vi "Setup manipulator (SubVI).vi"(0 "Release?":bool, 1 "G_upper bound":i32, 3 "M_lower bound":i32, 11 "error in (no error)":errorcluster, 12 "M_Encoder Ref In":T1, 14 "G_Encoder Ref In":T1) -> (15 "error out":errorcluster)   [LabVIEW 2017]
uses:
  <vilib>/myRIO/Instrument Drivers/Onboard IO/Encoder/typedefs/Encoder Reference.ctl
  <vilib>/myRIO/Common/Instrument Driver Framework/Utilities/typedefs/myRIO Generic Hardware Reference.ctl
  <vilib>/myRIO/Common/Instrument Driver Framework/Utilities/typedefs/Hardware Version Enum.ctl
  <vilib>/myRIO/Common/Instrument Driver Framework/Utilities/typedefs/myRIO v1.0 Reference.ctl
  <vilib>/myRIO/Common/Instrument Driver Framework/Utilities/typedefs/Generic FPGA Reference.ctl
  <vilib>/myRIO/Common/Instrument Driver Framework/myRIO v1.0/Encoder/typedefs/Encoder Channels Enum.ctl
  <vilib>/myRIO/Instrument Drivers/Onboard IO/DIO/typedefs/DIO Reference.ctl
  <vilib>/myRIO/Common/Instrument Driver Framework/myRIO v1.0/DIO/typedefs/DIO Channels List.ctl
  <vilib>/myRIO/Common/Instrument Driver Framework/myRIO v1.0/DIO/typedefs/DIO Channels Enum.ctl
  <vilib>/userdefined/High Color/nirio_resource_hc.ctl
  <vilib>/myRIO/Common/Instrument Driver Framework/Utilities/vis/Is FPGA Ref Available.vi
  <vilib>/myRIO/Common/Instrument Driver Framework/myRIO v1.0/DIO/vis/myRIO v1.1 Open DIO.vi
  <vilib>/myRIO/Instrument Drivers/Onboard IO/DIO/vis/Write.vi
  <vilib>/myRIO/Common/Instrument Driver Framework/Utilities/vis/Validate Channels.vi
  <vilib>/myRIO/Common/Instrument Driver Framework/myRIO v1.0/DIO/vis/myRIO v1.0 Reserve DIO.vi
  <vilib>/myRIO/Common/Instrument Driver Framework/myRIO v1.0/Resource Manager/vis/myRIO v1.0 Reserve Channel List.vi
  <vilib>/myRIO/Common/Instrument Driver Framework/myRIO v1.0/DIO/vis/myRIO v1.0 Build MUX Configuration DIO.vi
  <vilib>/myRIO/Common/Instrument Driver Framework/myRIO v1.0/Resource Manager/vis/myRIO v1.0 Reserve Channel.vi
  <vilib>/myRIO/Common/Instrument Driver Framework/myRIO v1.0/Resource Manager/vis/myRIO v1.0 Unreserve Channel.vi
  <vilib>/myRIO/Common/Instrument Driver Framework/myRIO v1.0/Resource Manager/vis/myRIO v1.0 Create Configuration List.vi
  <vilib>/myRIO/Common/Instrument Driver Framework/myRIO v1.0/Resource Manager/vis/myRIO v1.0 Build Mutex Name.vi
  <vilib>/Utility/error.llb/Error Cluster From Error Code.vi
  <vilib>/myRIO/Common/Instrument Driver Framework/myRIO v1.0/Encoder/vis/myRIO v1.0 Read Encoder.vi
  <vilib>/Utility/VariantDataType/GetNumericInfo.vi
  <vilib>/myRIO/Common/Instrument Driver Framework/myRIO v1.0/myRIO v1.1 Open.vi
  <vilib>/myRIO/Common/Instrument Driver Framework/Utilities/vis/IO Manager.vi
  <vilib>/myRIO/Common/Instrument Driver Framework/Utilities/vis/Configuration Manager.vi
  <vilib>/myRIO/Common/Instrument Driver Framework/myRIO v1.0/Resource Manager/vis/myRIO v1.0 Configure IO.vi
  <vilib>/myRIO/Common/Instrument Driver Framework/myRIO v1.0/myRIO v1.0 Close.vi
  <vilib>/myRIO/Common/Instrument Driver Framework/myRIO v1.0/DIO/vis/myRIO v1.0 Write DIO.vi
  <vilib>/myRIO/Express VI/Onboard IO/DO/DO Express VI.xnode
  <vilib>/myRIO/Instrument Drivers/Onboard IO/DIO/vis/myRIO DIO Open.xnode
  <vilib>/myRIO/Instrument Drivers/Onboard IO/Encoder/Encoder.lvlib
  <vilib>/myRIO/Instrument Drivers/Onboard IO/DIO/DIO.lvlib
panel:
  in  "stopG":bool
  out "G+":bool
  out "G enc val":i32
  out "M+":bool
  in  "stopM":bool
  out "M enc val":i32
  # "SET UP THE VALUES"
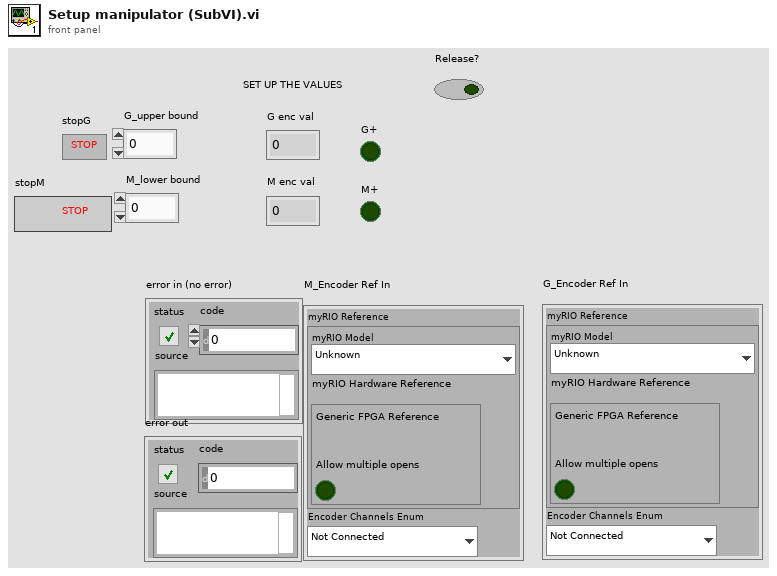
[diagram p1: front panel]
types:
  T1 = typedef "Encoder.lvlib/Encoder Reference.ctl" = cluster{"myRIO Reference":T2, "Encoder Channels Enum":T6}
  T2 = typedef "myRIO Generic Hardware Reference.ctl" = cluster{"myRIO Model":T3, "myRIO Hardware Reference":T4}
  T3 = typedef "Hardware Version Enum.ctl" = enum16{"Unknown", "myRIO-1900", "myRIO-1950", "roboRIO", "NI ELVIS RIO CM"}
  T4 = typedef "myRIO v1.0 Reference.ctl" = cluster{"Generic FPGA Reference":T5, "Allow multiple opens":bool}
  T5 = typedef "Generic FPGA Reference.ctl" = refnum<k20>
  T6 = typedef "Encoder Channels Enum.ctl" = enum16{"Not Connected", "C/ENC0", "C/ENC1", "A/ENC", "B/ENC", "DIO/ENC0", "DIO/ENC1", "DIO/ENC2", "DIO/ENC3", "DIO/ENC4"}
  T7 = typedef "DIO.lvlib/DIO Reference.ctl" = cluster{"myRIO Reference":T2, "DIO Channels List":T8}
  T8 = typedef "DIO Channels List.ctl" = T9[]
  T9 = typedef "DIO Channels Enum.ctl" = enum16{"Not Connected", "C/DIO0", "C/DIO1", "C/DIO2", "C/DIO3", "C/DIO4", "C/DIO5", "C/DIO6", "C/DIO7", "A/DIO0", "A/DIO1", "A/DIO2", "A/DIO3", "A/DIO4", "A/DIO5", "A/DIO6", "A/DIO7", "A/DIO8", "A/DIO9", "A/DIO10", "A/DIO11", "A/DIO12", "A/DIO13", "A/DIO14", "A/DIO15", "B/DIO0", "B/DIO1", "B/DIO2", "B/DIO3", "B/DIO4", "B/DIO5", "B/DIO6", "B/DIO7", "B/DIO8", "B/DIO9", "B/DIO10", "B/DIO11", "B/DIO12", "B/DIO13", "B/DIO14", "B/DIO15", "LED0", "LED1", "LED2", "LED3", "Button0", "DIO/DIO0", "DIO/DIO1", "DIO/DIO2", "DIO/DIO3", "DIO/DIO4", "DIO/DIO5", "DIO/DIO6", "DIO/DIO7", "DIO/DIO8", "DIO/DIO9", "SPI/CS0", "SPI/CS1", "SPI/CS2", "SPI/CS3", "LED RADIO (Green)", "LED RADIO (Red)", "LED COMM (Green)", "LED COMM (Red)", "LED MODE (Green)", "LED MODE (Red)"}
  T10 = typedef "nirio_resource_hc.ctl" = tag
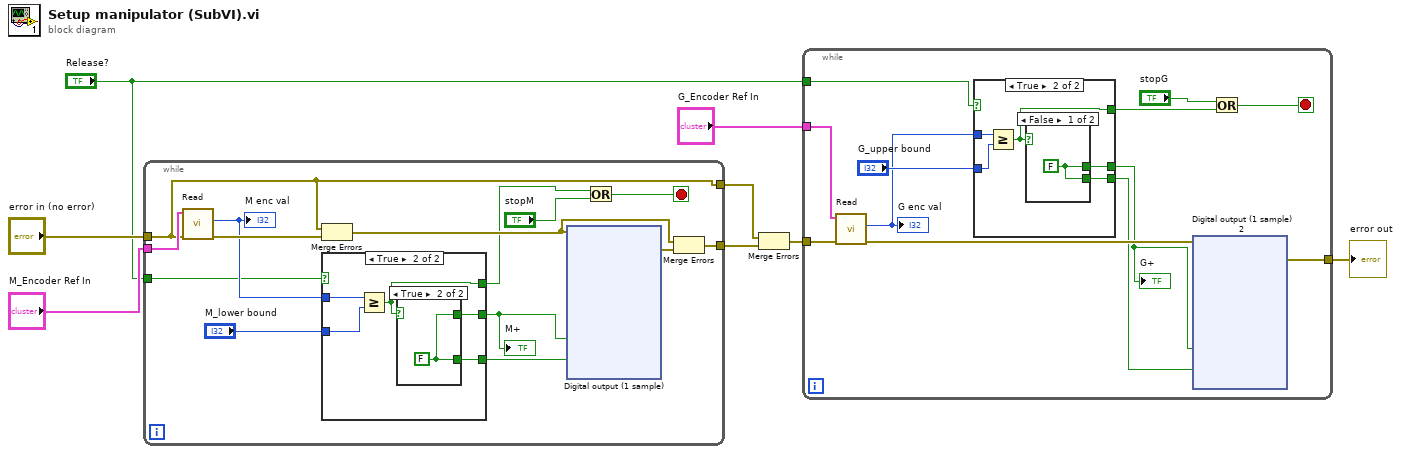
[diagram p0: block diagram]
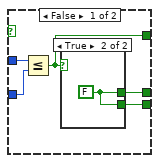
[diagram p2: hidden frame]
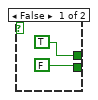
[diagram p3: hidden frame]
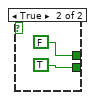
[diagram p4: hidden frame]
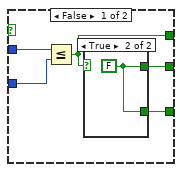
[diagram p5: hidden frame]
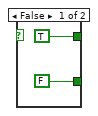
[diagram p6: hidden frame]
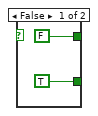
[diagram p7: hidden frame]
diagram:
  n1 = while {
    tunnel: "error in (no error)" -> [w19]
    tunnel: [w19] -> w7
    tunnel: [w21] -> w6
    tunnel: "M_Encoder Ref In" -> [w20]
    tunnel: "Release?" -> [w12]
    stop <- w16 stop-if-true
    n2 = call <vilib>:"Read.vi"("error in (no error)"=w19, "Encoder Ref In"=w20) -> ("error out"=w18:errorcluster, "Counter Value"=w17:i32)  [unwired: 5 in, 3 out]
    "M enc val" <- w17
    n3 = Merge Errors(w19, w18) -> (w13:errorcluster)
    n4 = case shown="True" w12 {
      tunnel: "M_lower bound" -> [w27 w35]
      tunnel: [w23 w31] -> w11
      tunnel: w17 -> [w26 w34]
      tunnel: [w25 w32] -> w10
      tunnel: [w24 w33] -> w9
      frame False {
        n5 = Less Or Equal?(x=w26, y=w27) -> (x <= y?=w23:bool)
        n6 = case shown="True" w23 {
          tunnel: [TRUE w30] -> w25
          tunnel: [FALSE w30] -> w24
          frame False {
          }
          frame True {
            w30 = FALSE
          }
        }
      }
      frame True {
        n7 = Greater Or Equal?(x=w34, y=w35) -> (x >= y?=w31:bool)
        n8 = case shown="True" w31 {
          tunnel: [TRUE ("M- (B/DIO6 (Pin 23))") w38] -> w33
          tunnel: [FALSE ("M- (B/DIO6 (Pin 23))") w38] -> w32
          frame False {
          }
          frame True {
            w38 = FALSE
          }
        }
      }
    }
    "M+" <- w10
    n9 = xnode "Digital output (1 sample)"("M+ (B/DIO5 (Pin 21))"=w10, "M- (B/DIO6 (Pin 23))"=w9, "error in (no error)"=w13) -> ("error out"=w14:errorcluster)
    n10 = Or(x=w11, y="stopM") -> (x .or. y?=w16:bool)
    n11 = Merge Errors(w13, w14) -> (w21:errorcluster)
  }
  n12 = Merge Errors(w7, w6) -> (w4:errorcluster)
  n13 = while {
    tunnel: w4 -> [w83]
    tunnel: [w78] -> w3
    tunnel: "G_Encoder Ref In" -> [w82]
    tunnel: "Release?" -> [w77]
    stop <- w80 stop-if-true
    n14 = call <vilib>:"Read.vi"("error in (no error)"=w83, "Encoder Ref In"=w82) -> ("error out"=w84:errorcluster, "Counter Value"=w85:i32)  [unwired: 5 in, 3 out]
    "G enc val" <- w85
    n15 = case shown="True" w77 {
      tunnel: "G_upper bound" -> [w91 w99]
      tunnel: w85 -> [w90 w98]
      tunnel: [w87 w95] -> w79
      tunnel: [w89 w96] -> w76
      tunnel: [w88 w97] -> w75
      frame False {
        n16 = Less Or Equal?(x=w90, y=w91) -> (x <= y?=w87:bool)
        n17 = case shown="True" w87 {
          tunnel: [TRUE w94] -> w89
          tunnel: [FALSE w94] -> w88
          frame False {
          }
          frame True {
            w94 = FALSE
          }
        }
      }
      frame True {
        n18 = Greater Or Equal?(x=w98, y=w99) -> (x >= y?=w95:bool)
        n19 = case shown="False" w95 {
          tunnel: [w100 TRUE] -> w97
          tunnel: [w100 FALSE] -> w96
          frame False {
            w100 = FALSE
          }
          frame True {
          }
        }
      }
    }
    "G+" <- w76
    n20 = xnode "Digital output (1 sample) 2"("G- (B/DIO7 (Pin 25))"=w76, "G+ (B/DIO13 (Pin 26))"=w75, "error in (no error)"=w84) -> ("error out"=w78:errorcluster)
    n21 = Or(x="stopG", y=w79) -> (x .or. y?=w80:bool)
  }
  "error out" <- w3
